vi "Write Digital Out.vi"(8 "error in (no error)":errorcluster, 10 "Digital Out":bool[](array[boolean]), 11 "DigitalIO in":refnum<class "DigitalIO.lvclass">) -> (0 "error out":errorcluster, 3 "DigitalIO out":refnum<class "DigitalIO.lvclass">)   [LabVIEW 2018, in "DigitalIO.lvlib" / "DigitalIO.lvclass"]
uses:
  DigitalIO.lvclass
  DigitalIO.lvclass/DigitalIO.ctl
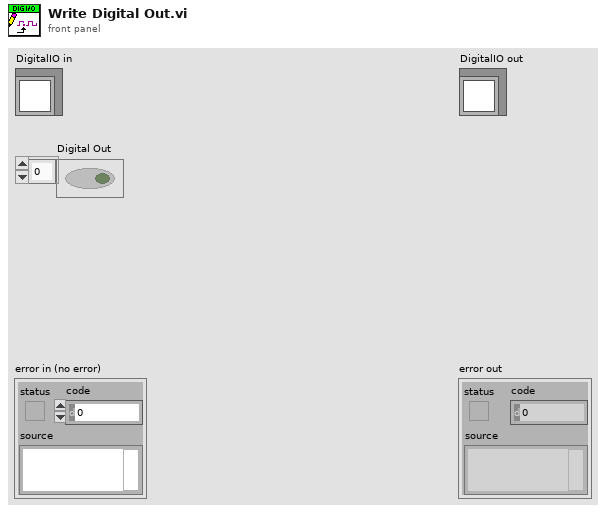
[diagram p1: front panel]
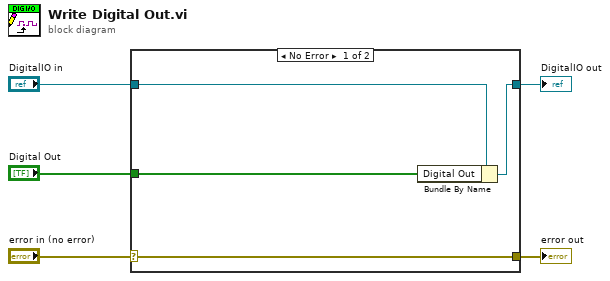
[diagram p0: block diagram]
diagram:
  n1 = case shown="No Error" "error in (no error)" {
    selector: "error in (no error)" -> [w9 w10]
    tunnel: [w9 w10] -> w4
    tunnel: [w7 w11] -> w2
    tunnel: "DigitalIO in" -> [w8 w11]
    tunnel: "Digital Out" -> [w6 _]
    frame No Error {
      n2 = Bundle By Name(cluster=w8, "Digital Out"=w6) -> (w7:refnum<class "DigitalIO.lvclass">)
    }
    frame Error {
    }
  }
  "error out" <- w4
  "DigitalIO out" <- w2
